vi "Configure DO.vi"(8 "error in (no error)":errorcluster, 10 "Enable Line":tag, 11 "DAQ HVPS in":refnum<class "DAQ HVPS.lvclass">) -> (0 "error out":errorcluster, 3 "DAQ HVPS out":refnum<class "DAQ HVPS.lvclass">)   [LabVIEW 2014, in "DAQ HVPS.lvclass"]
uses:
  DAQ HVPS.lvclass
  DAQ HVPS.lvclass/DAQ HVPS.ctl
  <vilib>/DAQmx/create/channels.llb/DAQmx Create Channel (DO-Digital Output).vi
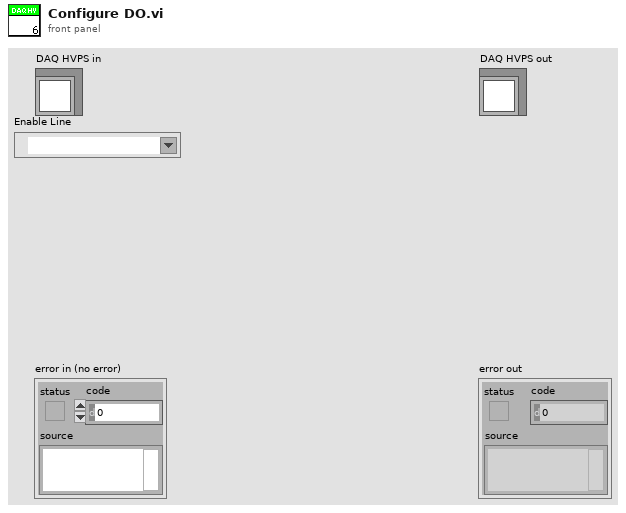
[diagram p1: front panel]
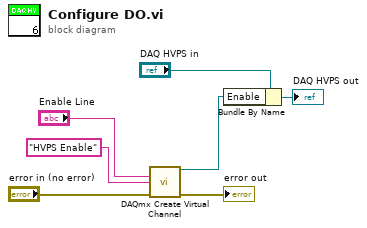
[diagram p0: block diagram]
diagram:
  n1 = call-poly <vilib>:"DAQmx Create Virtual Channel.vi"("lines"="Enable Line", "name to assign"="HVPS Enable", "error in"="error in (no error)") -> ("task out"=w2:refnum<k21>, "error out"=→"error out":errorcluster)  [unwired: 11 in]
  n2 = Bundle By Name(cluster="DAQ HVPS in", "Enable"=w2) -> (→"DAQ HVPS out":refnum<class "DAQ HVPS.lvclass">)
